vi "Global - Device.vi"() -> ()   [LabVIEW 2019]
panel:
  in  "Device":string[](array[string])
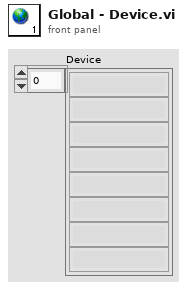
[diagram p1: front panel]
diagram:
